vi "9進階題-倒數碼表.vi"() -> ()   [LabVIEW 2019]
panel:
  out "倒數中":bool
  in  "開始":bool
  in  "Stop":bool
  in  "計時秒數(s)":u8
  out "Gauge":dbl(knob) max=4.0 scale=0.0..5.0
  # "按鍵「開始」後，碼表刻度數值變成「計時秒數」，開始倒數。\n時間到後，「倒數中」燈號熄滅。\n註：使用Property Node>>Scale>>Range>>Maximum可改變Gauge的秒數"
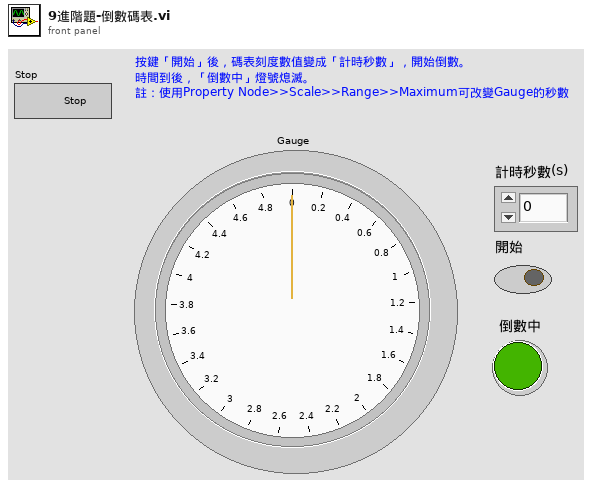
[diagram p1: front panel]
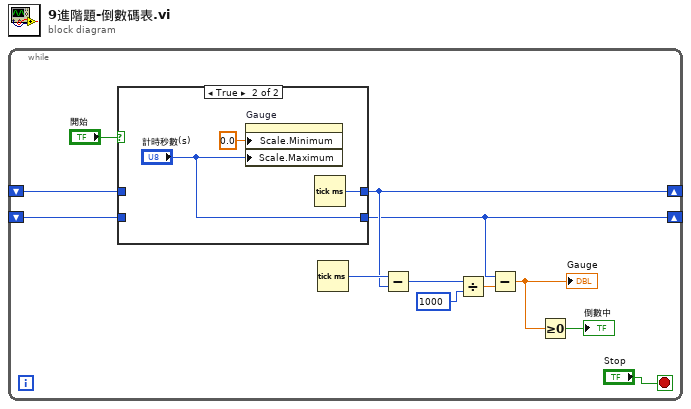
[diagram p0: block diagram]
diagram:
  n1 = while {
    shift-right: [w9] -> _
    shift-left: _ -> [w11]
    shift-right: [w4] -> _
    shift-left: _ -> [w5]
    stop <- "Stop" stop-if-true
    n2 = case shown="True" "開始" {
      tunnel: [w14 w17] -> w9
      tunnel: w11 -> [w14 _]
      tunnel: [w13 "計時秒數(s)"] -> w4
      tunnel: w5 -> [w13 _]
      frame False {
      }
      frame True {
        n3 = property on="Gauge" class="Knob (strict)"("Scale.Minimum"=0.0 ("Scale.Range:Minimum"), "Scale.Maximum"="計時秒數(s)") -> ()  [unwired: 2 in, 2 out]
        n4 = Tick Count (ms)() -> (millisecond timer value=w17:u32)
      }
    }
    n5 = Tick Count (ms)() -> (millisecond timer value=w10:u32)
    n6 = Subtract(x=w10, y=w9) -> (x-y=w7:u32)
    n7 = Divide(x=w7, y=u32 1000) -> (x/y=w3:dbl)
    n8 = Subtract(x=w4, y=w3) -> (x-y=w2:dbl)
    "Gauge" <- w2
    n9 = Greater Or Equal To 0?(x=w2) -> (x >= 0?=→"倒數中":bool)
  }
